vi "Walk Library.vi"(8 "error in (no error)":errorcluster, 11 "Library":refnum<vi>) -> (0 "error out":errorcluster, 3 "All VIs":set{path}(c389), 4 "Vimformation":map{path, T1}(c390), 5 "Library Out":refnum<vi>)   [LabVIEW 2020, in "vim-liner.lvlib"]
uses:
  vim-liner.lvlib
  vim-formation.ctl
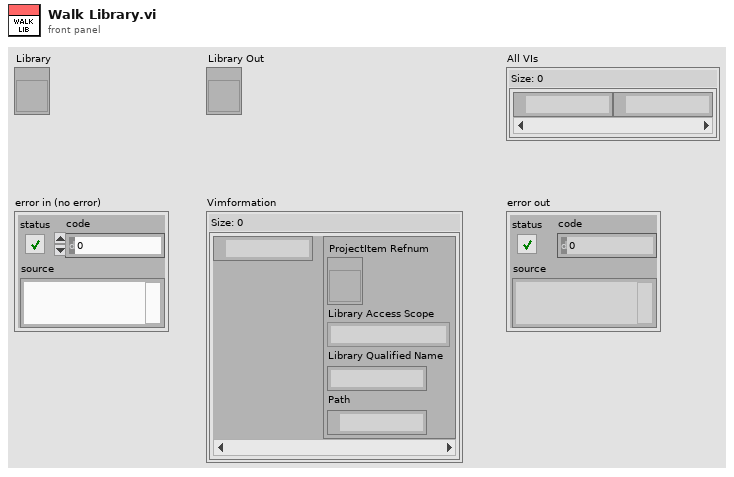
[diagram p1: front panel]
types:
  T1 = typedef "vim-liner.lvlib/vim-formation.ctl" = cluster{"ProjectItem Refnum":refnum<vi>, "Library Access Scope":enum32{"invalid scope", "public", "private", "protected", "community"}, "Library Qualified Name":string, "Path":path}
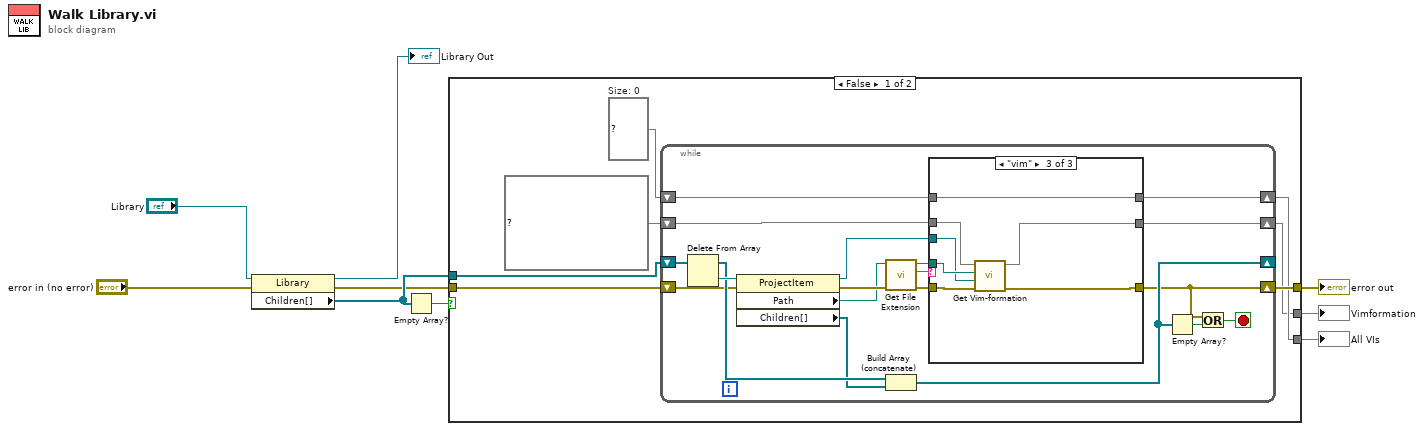
[diagram p0: block diagram]
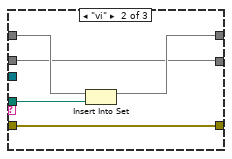
[diagram p3: hidden frame]
diagram:
  n1 = property class="Library"(reference="Library", error in="error in (no error)") -> (reference out=→"Library Out":refnum<vi>, error out=w7:errorcluster, "Children[]"=w8:refnum<vi>[])
  n2 = Empty Array?(array=w8) -> (empty?=w6:bool)
  n3 = case shown="False" w6 {
    tunnel: w7 -> [w15 w51]
    tunnel: w8 -> [w16 _]
    tunnel: [w14 w51] -> w9
    tunnel: [w12 _] -> w5
    tunnel: [w11 _] -> w4
    frame False {
      w13 = set{path} {}  # Size: 0
      n4 = while {
        shift-right: [w32] -> _
        shift-left: w16 -> [w35]
        shift-right: [w24] -> w14
        shift-left: w15 -> [w30]
        shift-right: [w20] -> w12
        shift-left: w13 -> [w21]
        shift-right: [w18] -> w11
        shift-left: map{path, T1} {} ("Vimformation") -> [w17]
        stop <- w25 stop-if-true
        n5 = Delete From Array(array=w35) -> (deleted portion=w34:refnum<vi>, array with subset deleted=w33:refnum<vi>[])  [unwired: 2 in]
        n6 = property class="ProjectItem"(reference=w34, error in=w30) -> (reference out=w19:refnum<vi>, error out=w29:errorcluster, "Path"=w22:path, "Children[]"=w23:refnum<vi>[])
        n7 = call <vilib>:"Get File Extension.vi"("error in (no error)"=w29, "file"=w22) -> ("error out"=w28:errorcluster, "lowercase file extension"=w27:string, "dup file"=w26:path)  [unwired: 5 in, 2 out]
        n8 = Build Array (concatenate)(w33, w23) -> (w32:refnum<vi>[])
        n9 = case shown="\"vim\"" w27 {
          tunnel: w28 -> [w38 w40 w49]
          tunnel: w26 -> [_ w43 w45]
          tunnel: [w38 w40 w48] -> w24
          tunnel: w21 -> [w37 w42 w50]
          tunnel: [w37 w41 w50] -> w20
          tunnel: w19 -> [_ _ w44]
          tunnel: [w36 w39 w47] -> w18
          tunnel: w17 -> [w36 w39 w46]
          frame Default {
          }
          frame "vi" {
            n10 = Insert Into Set(10:w43, 11:w42) -> (3:w41:set{path})  [unwired: 1 out]
          }
          frame "vim" {
            n11 = call "Get Vim-formation.vi"("error in (no error)"=w49, "ProjectItem Refnum"=w44, "Path"=w45, "Map in"=w46) -> ("error out"=w48:errorcluster, "Map out"=w47:map{path, T1})  [unwired: 6 in]
          }
        }
        n12 = Empty Array?(array=w32) -> (empty?=w31:bool)
        n13 = Or(x=w24, y=w31) -> (x .or. y?=w25:bool)
      }
    }
    frame True {
    }
  }
  "error out" <- w9
  "All VIs" <- w5
  "Vimformation" <- w4
